vi "thermistor.vi"() -> ()   [LabVIEW 2021]
uses:
  <vilib>/Utility/file.llb/Write Delimited Spreadsheet (string).vi
  <vilib>/express/express arith-compare/Formula/XNode/ExpressFormulaBlockNode.xnode
panel:
  in  "File Path":path
  out "Celsius":dbl
  out "Fahrenheit":dbl
  out "Kelvin":dbl
  in  "stop":bool
  in  "High Limit (F)":dbl
  in  "Low Limit (F)":dbl
  out "High":bool
  out "Low":bool
  out "Temperature (F)":dbl(slide) scale=32.0..212.0
  out "Temperature (C)":dbl(slide) scale=0.0..100.0
  out "Temperature (K)":dbl(slide) scale=273.0..373.0
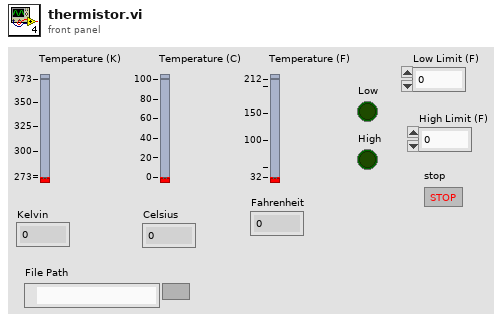
[diagram p1: front panel]
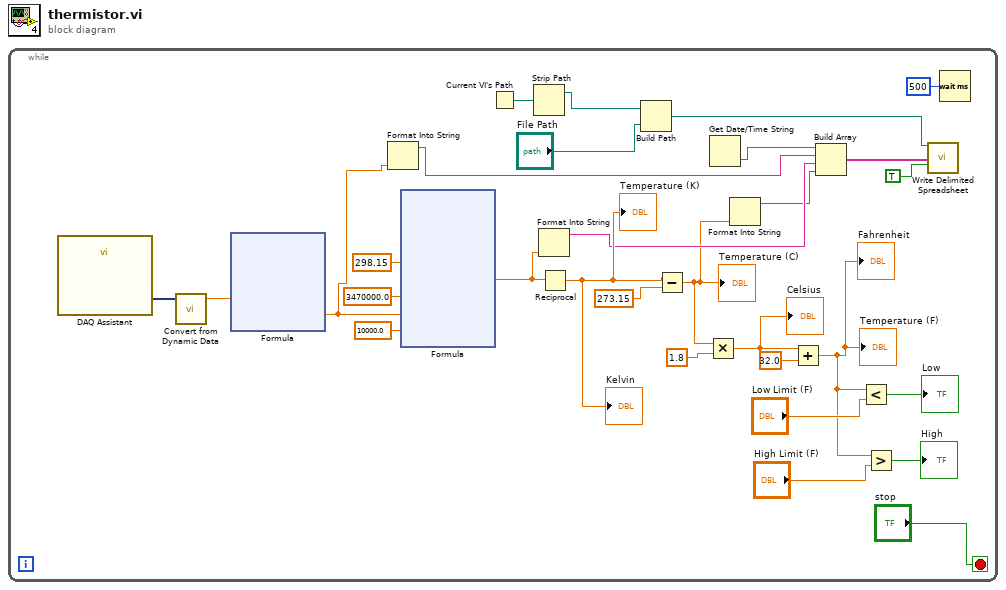
[diagram p0: block diagram]
diagram:
  n1 = while {
    stop <- "stop" stop-if-true
    n2 = call "DAQ Assistant"() -> ("data"=w19:dynamicdata)  [unwired: 17 in, 2 out]
    n3 = call "Convert from Dynamic Data"("Dynamic Data Type"=w19) -> ("Scalar"=w20:dbl)  [unwired: 3 in]
    n4 = xnode "Formula"("VR2"=w20) -> ("Result"=w8:dbl)  [unwired: 1 in, 1 out]
    n5 = Format Into String(w8) -> (resulting string=w7:string)  [unwired: 3 in, 1 out]
    n6 = xnode "Formula"("T0"=298.15, "B"=3470000.0, "Rt"=w8, "R0"=10000.0) -> ("Result"=w6:dbl)  [unwired: 1 in, 1 out]
    n7 = Current VI's Path() -> (path=w13:path)
    n8 = Strip Path(path=w13) -> (stripped path=w11:path)  [unwired: 1 out]
    n9 = Format Into String(w6) -> (resulting string=w5:string)  [unwired: 3 in, 1 out]
    n10 = Reciprocal(x=w6) -> (1/x=w17:dbl)
    "Temperature (K)" <- w17
    "Kelvin" <- w17
    n11 = Build Path(base path=w11, name or relative path="File Path") -> (appended path=w10:path)
    n12 = Subtract(x=w17, y=273.15) -> (x-y=w3:dbl)
    "Temperature (C)" <- w3
    n13 = Multiply(x=w3, y=1.8) -> (x*y=w15:dbl)
    "Celsius" <- w15
    n14 = Get Date/Time String() -> (time string=w9:string)  [unwired: 3 in, 1 out]
    n15 = Format Into String(w3) -> (resulting string=w4:string)  [unwired: 3 in, 1 out]
    n16 = Add(x=w15, y=32.0) -> (x+y=w16:dbl)
    "Temperature (F)" <- w16
    "Fahrenheit" <- w16
    n17 = Build Array(w9, w7, w5, w4) -> (w2:string[])
    n18 = Less?(x=w16, y="Low Limit (F)") -> (x < y?=→"Low":bool)
    n19 = Greater?(x=w16, y="High Limit (F)") -> (0:→"High":bool)
    n20 = call-poly <vilib>:"Write Delimited Spreadsheet.vi"("file path (dialog if empty)"=w10, "1D data"=w2, "append to file? (new file:F)"=TRUE) -> ()  [unwired: 11 in, 2 out]
    n21 = Wait (ms)(milliseconds to wait=u32 500) -> ()  [unwired: 1 out]
  }
